vi "locationsToTime.vi"(10 "Locations":dbl[](array[numeric]), 11 "time in":dbl[](array[numeric])) -> (3 "time out":dbl[](array[numeric]))   [LabVIEW 2014]
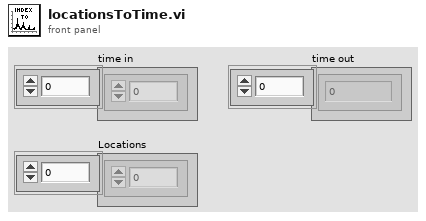
[diagram p1: front panel]
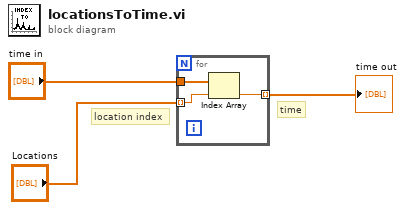
[diagram p0: block diagram]
diagram:
  # "time"
  # "location index"
  n1 = for {
    tunnel: "time in" -> [w6]
    tunnel: "Locations" -> [w5] mode=indexing
    tunnel: [w4] -> w2 mode=indexing
    n2 = Index Array(array=w6, index=w5) -> (element=w4:dbl)
  }
  "time out" <- w2
